vi "start.vi"(8 "error in (no error)":errorcluster, 11 "Analog_Input in":refnum<class "Analog_Input.lvclass">) -> (0 "error out":errorcluster, 3 "Analog_Input out":refnum<class "Analog_Input.lvclass">)   [LabVIEW 2013, in "Analog_Input.lvclass"]
uses:
  Analog_Input.lvclass
  Analog_Input.lvclass/Analog_Input.ctl
  Globals.vi
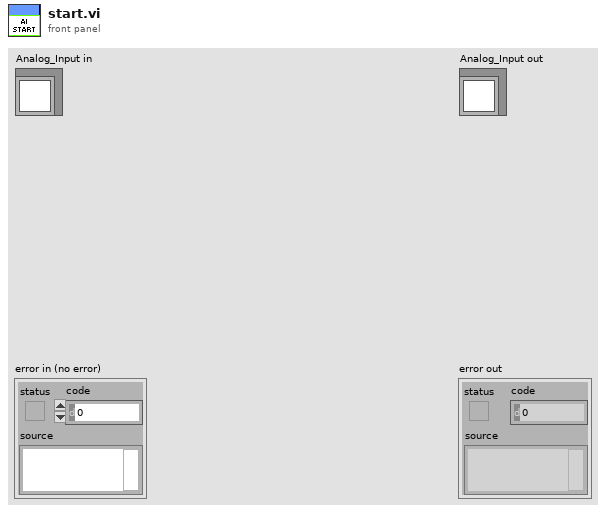
[diagram p1: front panel]
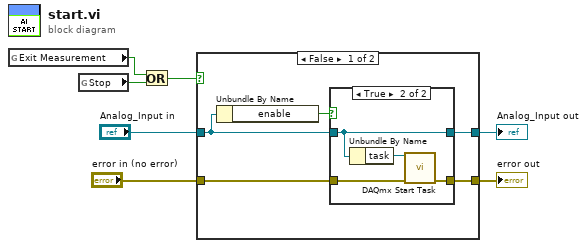
[diagram p0: block diagram]
diagram:
  n1 = global read "Globals.vi" "Exit Measurement"() -> (w3:bool)
  n2 = global read "Globals.vi" "Stop"() -> (w4:bool)
  n3 = Or(x=w3, y=w4) -> (x .or. y?=w2:bool)
  n4 = case shown="False" w2 {
    tunnel: [w10 w19] -> w7
    tunnel: [w8 w20] -> w5
    tunnel: "Analog_Input in" -> [w9 w20]
    tunnel: "error in (no error)" -> [w11 w19]
    frame False {
      n5 = Unbundle By Name(w9) -> ("enable"=w12:bool)
      n6 = case shown="True" w12 {
        tunnel: w11 -> [w13 w18]
        tunnel: [w13 w17] -> w10
        tunnel: w9 -> [w14 w15]
        tunnel: [w14 w15] -> w8
        frame False {
        }
        frame True {
          n7 = Unbundle By Name(w15) -> ("task"=w16:refnum<k21>)
          n8 = call <vilib>:"DAQmx Start Task.vi"("task/channels in"=w16, "error in"=w18) -> ("error out"=w17:errorcluster)  [unwired: 12 in, 1 out]
        }
      }
    }
    frame True {
    }
  }
  "error out" <- w7
  "Analog_Input out" <- w5
